vi "StopProgram.vi"(8 "error in (no error)":errorcluster, 11 "StepMotor in":refnum<class "StepMotor.lvclass">) -> (0 "error out":errorcluster, 3 "StepMotor out":refnum<class "StepMotor.lvclass">)   [LabVIEW 2010, in "StepMotor.lvclass"]
uses:
  StepMotor.lvclass
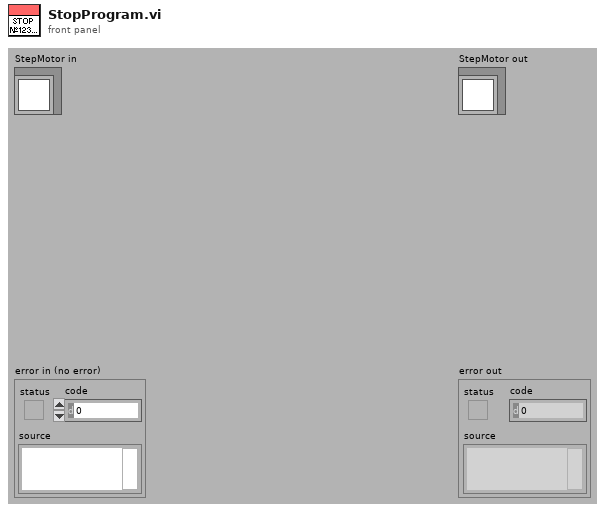
[diagram p1: front panel]
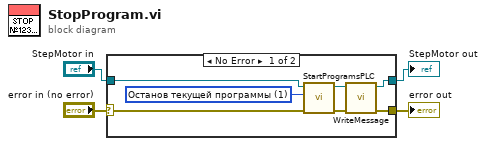
[diagram p0: block diagram]
diagram:
  n1 = case shown="No Error" "error in (no error)" {
    selector: "error in (no error)" -> [w7 w13]
    tunnel: [w5 w13] -> w3
    tunnel: [w6 w12] -> w1
    tunnel: "StepMotor in" -> [w8 w12]
    frame No Error {
      w9 = u16 1 items=["Запуск программы", "Останов текущей программы"] ("Тип запроса")
      n2 = call-dynamic "StartProgramsPLC.vi"("error in (no error)"=w7, "Тип запроса"=w9, "StepMotor in"=w8) -> ("error out"=w11:errorcluster, "StepMotor out"=w10:refnum<class "StepMotor.lvclass">)  [unwired: 7 in]
      n3 = call-dynamic "WriteMessage.vi"("error in (no error)"=w11, "StepMotor in"=w10) -> ("error out"=w5:errorcluster, "StepMotor out"=w6:refnum<class "StepMotor.lvclass">)  [unwired: 8 in]
    }
    frame Error {
    }
  }
  "error out" <- w3
  "StepMotor out" <- w1
